vi "ParseXBee.vi"(2 "XBee String":string) -> (0 "Bump 1":bool, 5 "Red":dbl, 6 "Blue":dbl, 7 "Green":dbl)   [LabVIEW 2012]
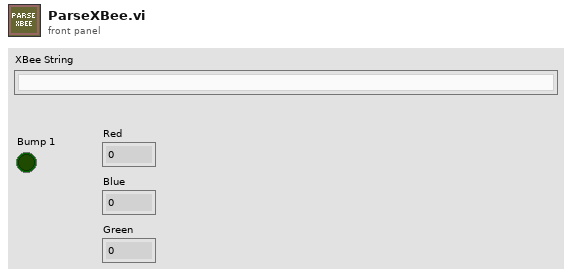
[diagram p1: front panel]
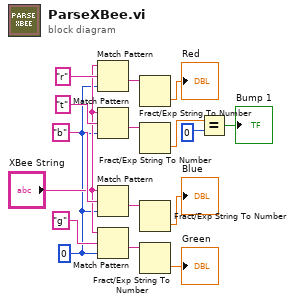
[diagram p0: block diagram]
diagram:
  w1 = 0 ("offset (0)")
  n1 = Match Pattern(string="XBee String", regular expression="r", offset (0)=w1) -> (after substring=w12:string)  [unwired: 3 out]
  n2 = Match Pattern(string="XBee String", regular expression="t", offset (0)=w1) -> (after substring=w9:string)  [unwired: 3 out]
  n3 = Match Pattern(string="XBee String", regular expression="b", offset (0)=w1) -> (after substring=w10:string)  [unwired: 3 out]
  n4 = Match Pattern(string="XBee String", regular expression="g", offset (0)=w1) -> (after substring=w11:string)  [unwired: 3 out]
  n5 = Fract/Exp String To Number(string=w12) -> (number=→"Red":dbl)  [unwired: 3 in, 1 out]
  n6 = Fract/Exp String To Number(string=w9) -> (number=w7:dbl)  [unwired: 3 in, 1 out]
  n7 = Fract/Exp String To Number(string=w10) -> (number=→"Blue":dbl)  [unwired: 3 in, 1 out]
  n8 = Fract/Exp String To Number(string=w11) -> (number=→"Green":dbl)  [unwired: 3 in, 1 out]
  n9 = Equal?(x=w7, y=0) -> (x = y?=→"Bump 1":bool)
